vi "Get Velocity.vi"(4 "error in (no error)":errorcluster, 5 "Wait before read (0ms)":u32, 6 "Axis (1)":i32=1 min=1 max=3, 7 "VISA resource name":refnum<visa-resource-name>) -> (0 "error out":errorcluster, 2 "Velocity (units/s)":dbl format="%.4g", 3 "VISA resource name out":refnum<visa-resource-name>)   [LabVIEW 2011, in "Newport ESP301.lvlib"]
doc: "Reads the velocity value for an axis."
uses:
  Newport ESP301.lvlib
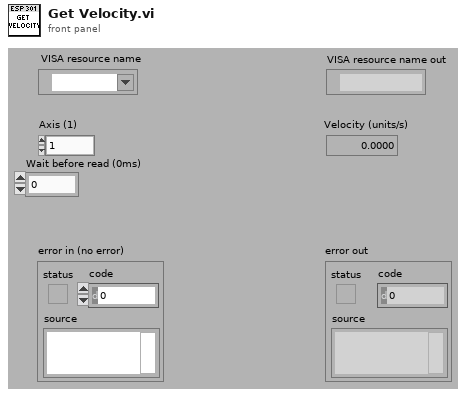
[diagram p1: front panel]
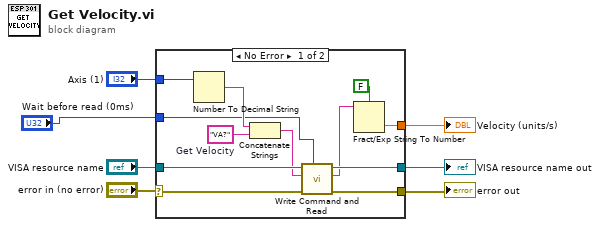
[diagram p0: block diagram]
diagram:
  n1 = case shown="No Error" "error in (no error)" {
    selector: "error in (no error)" -> [w16 w21]
    tunnel: [w18 w21] -> w7
    tunnel: "VISA resource name" -> [w19 w20]
    tunnel: [w17 w20] -> w6
    tunnel: [w14 _] -> w3
    tunnel: "Axis (1)" -> [w11 _]
    tunnel: "Wait before read (0ms)" -> [w8 _]
    frame No Error {
      w13 = "VA?"  # Get Velocity
      n2 = Number To Decimal String(number=w11) -> (decimal integer string=w12:string)  [unwired: 1 out]
      n3 = Concatenate Strings(w12, w13) -> (w10:string)
      n4 = call "Write Command and Read.vi"("Wait before read (0ms)"=w8, "error in (no error)"=w16, "Command"=w10, "VISA resource name"=w19) -> ("error out"=w18:errorcluster, "Returned string"=w15:string, "VISA resource name out"=w17:refnum<visa-resource-name>)  [unwired: 1 in, 2 out]
      n5 = Fract/Exp String To Number(use system decimal point (T)=FALSE ("utiliser le séparateur décimal du système (V)"), string=w15) -> (number=w14:dbl)  [unwired: 3 out]
    }
    frame Error {
    }
  }
  "error out" <- w7
  "VISA resource name out" <- w6
  "Velocity (units/s)" <- w3
